vi "Add Capabilities.vi"(8 "error in (no error)":errorcluster, 10 "Capabilities":string[](array[string]), 11 "NodeDiscovery in":refnum<class "NodeDiscovery.lvclass">) -> (0 "error out":errorcluster, 3 "NodeDiscovery out":refnum<class "NodeDiscovery.lvclass">)   [LabVIEW 2020, in "Vecto.lvlib" / "NodeDiscovery.lvclass"]
uses:
  NodeDiscovery.lvclass
  NodeDiscovery.lvclass/NodeDiscovery.ctl
  Capabilities Action.ctl
  Capabilities Update Data.ctl
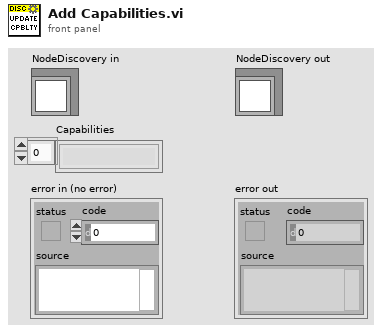
[diagram p1: front panel]
types:
  T1 = typedef "Vecto.lvlib/NodeDiscovery.lvclass/Capabilities Update Data.ctl" = cluster{"Action":T2, "Capabilities":string[]}
  T2 = typedef "Vecto.lvlib/NodeDiscovery.lvclass/Capabilities Action.ctl" = enum16{"Add", "Remove", "Clear"}
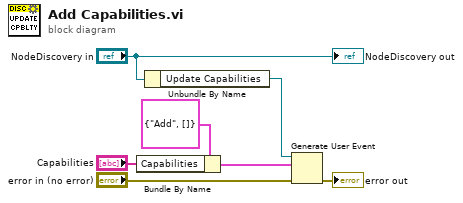
[diagram p0: block diagram]
diagram:
  n1 = Bundle By Name(cluster=T1 {"Action"=enum."Add", "Capabilities"=[]} ("Capabilities Update Data"), "Capabilities"="Capabilities") -> (w4:T1)
  n2 = Unbundle By Name("NodeDiscovery in") -> ("Update Capabilities"=w3:refnum<user-event>)
  n3 = Generate User Event(user event=w3, event data cluster=w4, error in="error in (no error)") -> (error out=→"error out":errorcluster)  [unwired: 1 in, 1 out]
  "NodeDiscovery out" <- "NodeDiscovery in"
